vi "Handle mouse enter.vi"(8 "error in (no error)":errorcluster, 11 "String dropdown D Element in":refnum<class "String dropdown D Element.lvclass">) -> (0 "error out":errorcluster, 2 "Active cursor":u16, 3 "String dropdown D Element out":refnum<class "String dropdown D Element.lvclass">)   [LabVIEW 2020, in "D Datagrid Library.lvlib" / "String dropdown D Element.lvclass"]
doc: "Sets the mouseover cursor for this element. Override this VI for each child that needs a custom (non-automatic) cursor."
uses:
  String dropdown D Element.lvclass
  String dropdown D Element.lvclass/String dropdown D Element.ctl
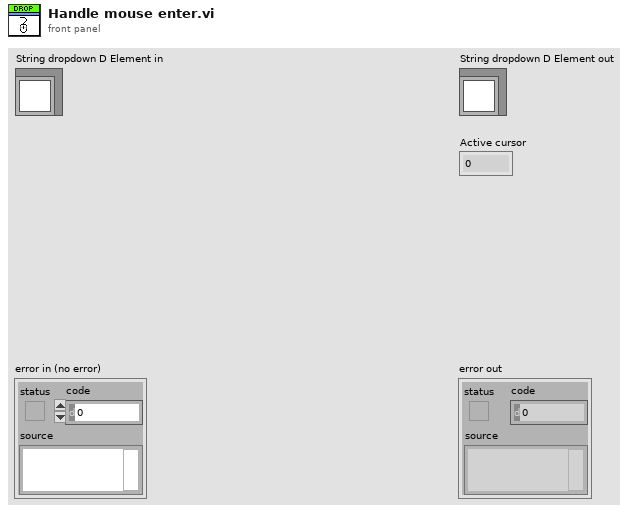
[diagram p1: front panel]
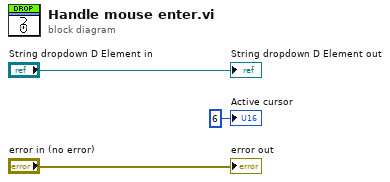
[diagram p0: block diagram]
diagram:
  "error out" <- "error in (no error)"
  "String dropdown D Element out" <- "String dropdown D Element in"
  "Active cursor" <- u16 6 ("Active cursor")
